vi "Send Start VST.vi"(7 "Message Priority (Normal)":T2=enum."Normal", 8 "error in (no error)":errorcluster, 10 "VST Config":T1={"Samples to Read per Block"=33554432, "IQ rate (S/s)"=1250000000.0, "Carrier Frequency (Hz)"=1000000000.0, "Reference Level (dBm)"=0.0, "Resource Name"="RFSA", "Clock Source"="OnboardClock", "Host DMA Buffer Size"=2000000000} {"Host DMA Buffer Size" format="%.0p"; "Reference Level (dBm)" format="%.2f"; "Carrier Frequency (Hz)" format="%#.3p"; "IQ rate (S/s)" format="%#.3p"; "Samples to Read per Block" min=1 format="%.0p"}, 11 "Message Enqueuer":refnum<class "Message Enqueuer.lvclass">) -> (0 "error out":errorcluster, 3 "Message Enqueuer out":refnum<class "Message Enqueuer.lvclass">)   [LabVIEW 2020, in "Application Manager.lvlib" / "Start VST Msg.lvclass"]
doc: "This VI sends the message to an actor."
uses:
  Start VST Msg.lvclass
  <vilib>/ActorFramework/Message Enqueuer/Message Enqueuer.lvclass
  <vilib>/ActorFramework/Message Enqueuer/Message Priority.ctl
  RFSA DAQ/RFSA DAQ/Configure VST.ctl
  C:/Program Files/National Instruments/LabVIEW 2025/vi.lib/ActorFramework/Message/Message.lvclass
  Start VST Msg.lvclass/Start VST Msg.ctl
  <vilib>/ActorFramework/Message Enqueuer/Message Enqueuer.lvclass/Message Enqueuer.ctl
  <vilib>/ActorFramework/Message Priority Queue/Priority Enqueue.vi
  RFSA DAQ/RFSA DAQ/RFSA DAQ.lvclass
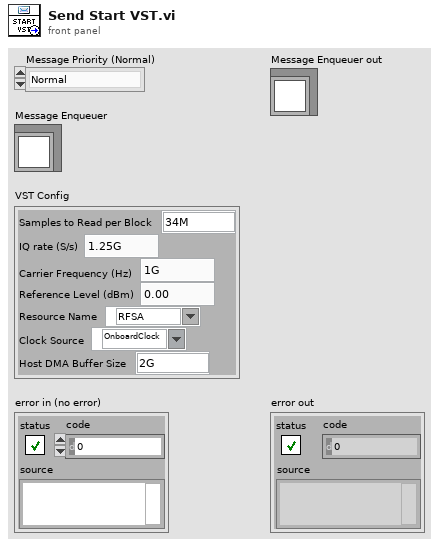
[diagram p1: front panel]
types:
  T1 = typedef "RFSA DAQ.lvlib/RFSA DAQ.lvclass/Configure VST.ctl" = cluster{"Samples to Read per Block":i32, "IQ rate (S/s)":dbl, "Carrier Frequency (Hz)":dbl, "Reference Level (dBm)":dbl, "Resource Name":refnum<k15>, "Clock Source":refnum<k15>, "Host DMA Buffer Size":i64}
  T2 = typedef "Actor Framework.lvlib/Message Enqueuer.lvclass/Message Priority.ctl" = enum16{"Low", "Normal", "High"}
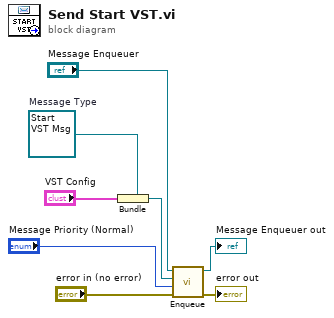
[diagram p0: block diagram]
diagram:
  w5 = refnum<class "Start VST Msg.lvclass"> refnum  # Message Type
  n1 = Bundle(cluster=w5, "VST Config") -> (w4:refnum<class "Start VST Msg.lvclass">)
  n2 = call <vilib>:"Enqueue.vi"("error in (no error)"="error in (no error)", "Message Priority (Normal)"="Message Priority (Normal)", "Message"=w4, "Message Enqueuer in"="Message Enqueuer") -> ("error out"=→"error out":errorcluster, "Message Enqueuer out"=→"Message Enqueuer out":refnum<class "Message Enqueuer.lvclass">)  [unwired: 6 in]
